vi "FTW-Actor-InitializeLogger.vi"(0 "FTW Actor Instance Type":refnum<class "FTW-ActorInstance.lvclass">, 7 "Actor Instance Configuration":string, 11 "error in":errorcluster) -> (4 "FTW Actor Instance":refnum<class "FTW-ActorInstance.lvclass">, 15 "error out":errorcluster)   [LabVIEW 2015, in "FTW-ActorInstance.lvclass"]
uses:
  FTW-ActorInstance.lvclass
  FTW-ActorInstance.lvclass/FTW-ActorInstance.ctl
  JSON/core/FTW-JSON-Core-EncodingFlags.vi
  JSON/FTW-JSON-Parse.vi
  Reflection/FTW-Reflection-Type.vi
  CodeGen/JSON Deserialize/FTW-JSON-Core-GetFlattenedValue.vi
  CodeGen/JSON Deserialize/FTW-JSON-Deserialize.xnode
  Ether/FTW-Ether.lvclass
panel:
  # "Inputs"
  # "Outputs"
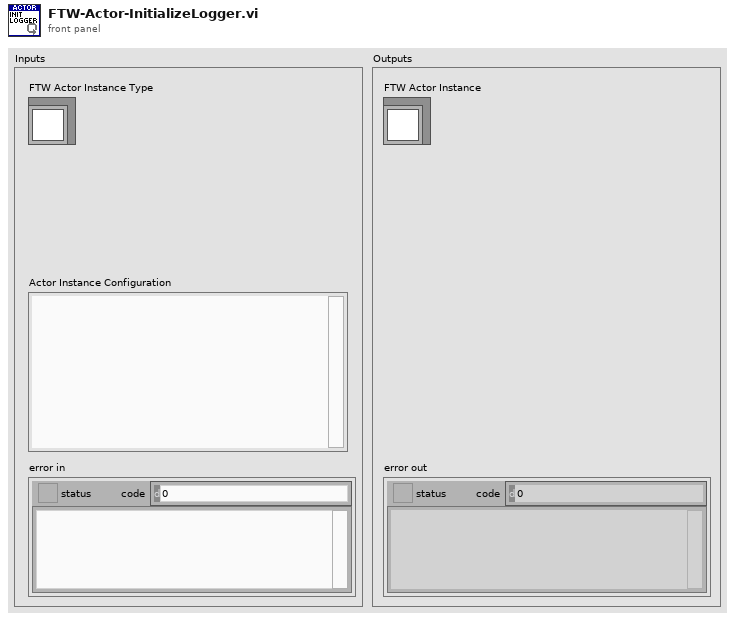
[diagram p1: front panel]
types:
  T1 = cluster{"LoggerAddress":string, "DebugEnableJobLogging":bool, "DebugEnableInboxLogging":bool}
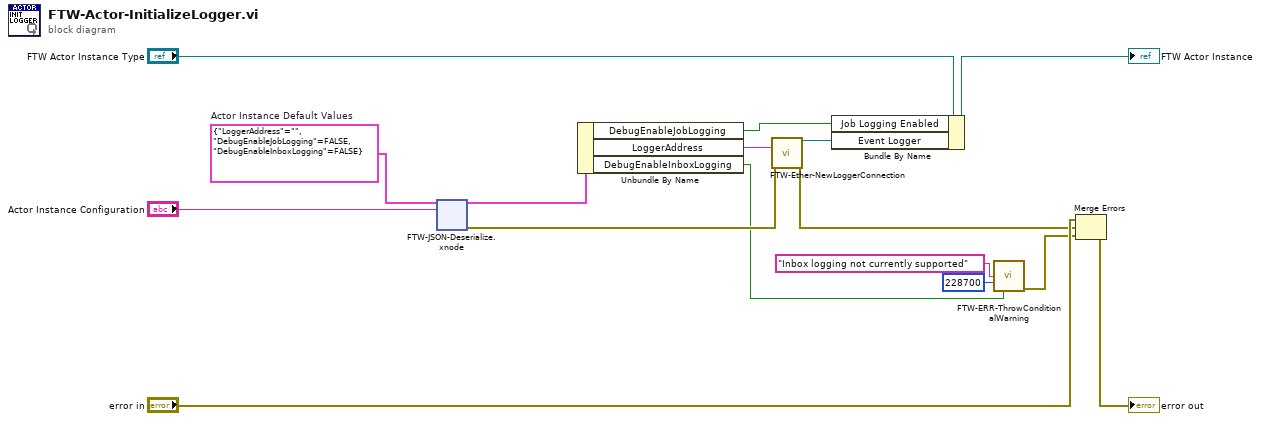
[diagram p0: block diagram]
diagram:
  w1 = T1 {"LoggerAddress"="", "DebugEnableJobLogging"=FALSE, "DebugEnableInboxLogging"=FALSE}  # Actor Instance Default Values
  n1 = xnode "FTW-JSON-Deserialize.xnode"("Type and Defaults"=w1, "JSON String"="Actor Instance Configuration") -> ("Values"=w14:T1, "error out"=w13:errorcluster)  [unwired: 1 in]
  n2 = Unbundle By Name(w14) -> ("DebugEnableJobLogging"=w11:bool, "LoggerAddress"=w2:string, "DebugEnableInboxLogging"=w4:bool)
  n3 = call "FTW-Ether-NewLoggerConnection.vi"("Logger Address"=w2, "error in"=w13) -> ("Event Logger Connection"=w12:refnum<class "FTW-Logger.lvclass">, "error out"=w3:errorcluster)  [unwired: 12 in]
  n4 = Bundle By Name(cluster="FTW Actor Instance Type", "Job Logging Enabled"=w11, "Event Logger"=w12) -> (→"FTW Actor Instance":refnum<class "FTW-ActorInstance.lvclass">)
  n5 = call "FTW-ERR-ThrowConditionalWarning.vi"("Warning Message"="Inbox logging not currently supported", "Error Code"=228700, "Throw?"=w4) -> ("error out"=w5:errorcluster)  [unwired: 12 in]
  n6 = Merge Errors("error in", w3, w5) -> (→"error out":errorcluster)
